vi "TextFit_Fill in Character Array.vi"(8 "Error":errorcluster, 11 "Character Array":T1[](array[typedef])) -> (0 "Error Out":errorcluster, 3 "Character Array Out":T1[](array[typedef]))   [LabVIEW 2014]
doc: "Calculates the pixel with of each character and sorts array by priority"
uses:
  Controls/Cluster/Cluster_Character Size and Priority Data.ctl
  Controls/String_Picture/String Char Normal.ctl
  Controls/Enum/ENUM_Font Size Select.ctl
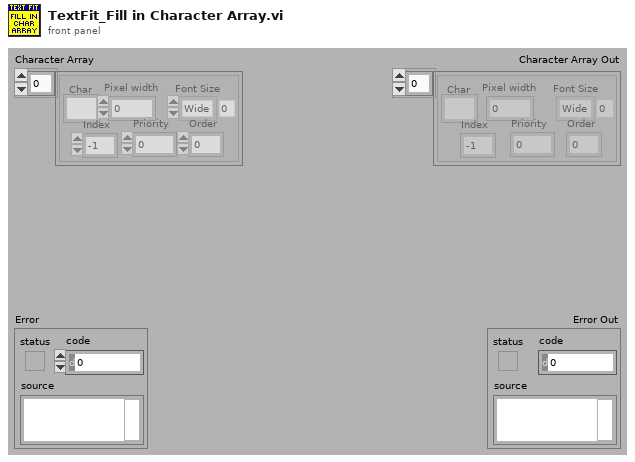
[diagram p1: front panel]
types:
  T1 = typedef "Cluster_Character Size and Priority Data.ctl" = cluster{"Char":T2, "Font Size":T3, "Pixel width":i32, "Priority":i32, "Order":i32, "Index":i32}
  T2 = typedef "String Char Normal.ctl" = string
  T3 = typedef "ENUM_Font Size Select.ctl" = enum16{"Wide", "Med", "Thin"}
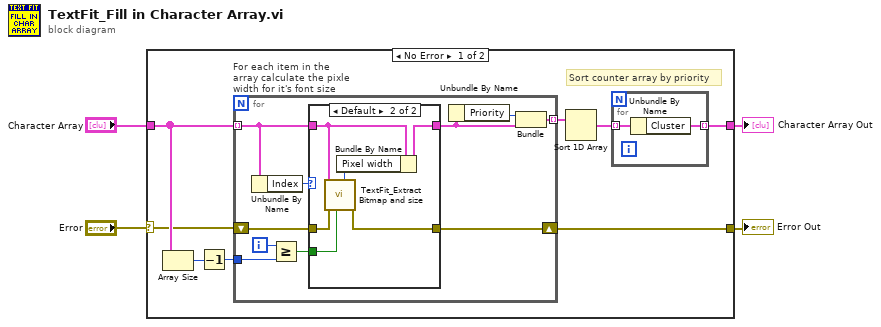
[diagram p0: block diagram]
diagram:
  n1 = case shown="No Error" "Error" {
    selector: "Error" -> [w5 w34]
    tunnel: [w12 w33] -> w4
    tunnel: [w9 w34] -> w3
    tunnel: "Character Array" -> [w8 w33]
    frame No Error {
      # "Sort counter array by priority"
      n2 = Array Size(array=w8) -> (size(s)=w7:i32)
      n3 = Decrement(x=w7) -> (x-1=w6:i32)
      n4 = for "For each item in the array calculate the pixle width for it's font size" {
        shift-right: [w20] -> w9
        shift-left: w5 -> [w24]
        tunnel: w8 -> [w19] mode=indexing
        tunnel: [w21] -> w10 mode=indexing
        tunnel: w6 -> [w15]
        i -> [w17]
        n5 = Unbundle By Name(w19) -> ("Index"=w18:i32)
        n6 = Greater Or Equal?(x=w17, y=w15) -> (x >= y?=w16:bool)
        n7 = case shown="Default" w18 {
          tunnel: w24 -> [w25 w31]
          tunnel: w19 -> [w26 w28]
          tunnel: [w26 w32] -> w22
          tunnel: [w25 w30] -> w20
          tunnel: w16 -> [_ w29]
          frame -1 {
          }
          frame Default {
            n8 = call "TextFit_Extract Bitmap and size.vi"("Last Character"=w29, "Error"=w31, "Character Cluster"=w28) -> ("Error Out"=w30:errorcluster, "Size Out"=w27:i32)  [unwired: 6 in, 1 out]
            n9 = Bundle By Name(cluster=w28, "Pixel width"=w27) -> (w32:T1)
          }
        }
        n10 = Unbundle By Name(w22) -> ("Priority"=w23:i32)
        n11 = Bundle("Priority"=w23, "Cluster"=w22) -> (w21:cluster{"Priority":i32, "Cluster":T1})  [unwired: 1 in]
      }
      n12 = Sort 1D Array(array=w10) -> (sorted array=w11:cluster{"Priority":i32, "Cluster":T1}[])
      n13 = for {
        tunnel: w11 -> [w14] mode=indexing
        tunnel: [w13] -> w12 mode=indexing
        n14 = Unbundle By Name(w14) -> ("Cluster"=w13:T1)
      }
    }
    frame Error {
    }
  }
  "Character Array Out" <- w4
  "Error Out" <- w3
